vi "SW_Fire_TTL_during_calibration_2.vi"(8 "error in (no error)":errorcluster, 9 "VISA resource in":refnum<visa-resource-name>="Tracker", 10 "Port to fire":u16(ring)=1 items=["Out 1"=1, "Out 2"=2, "Out 3"=4, "Out 4"=8], 11 "TTL pulse length, ms":dbl=250.0 format="%#_13g") -> (0 "error out":errorcluster, 1 "VISA resource out":refnum<visa-resource-name>="Tracker", 3 "Time spent to process command, ms":dbl)   [LabVIEW 2018, in "Tracker.lvlib"]
doc: "Fires TTL High to the TTL2 output for ~250 ms (default)."
uses:
  Tracker.lvlib
  <vilib>/Instr/_visa.llb/VISA Flush IO Buffer Mask.ctl
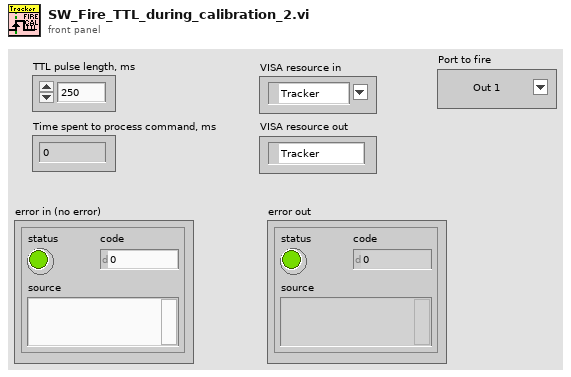
[diagram p1: front panel]
types:
  T1 = typedef "VISA Flush IO Buffer Mask.ctl" = u16
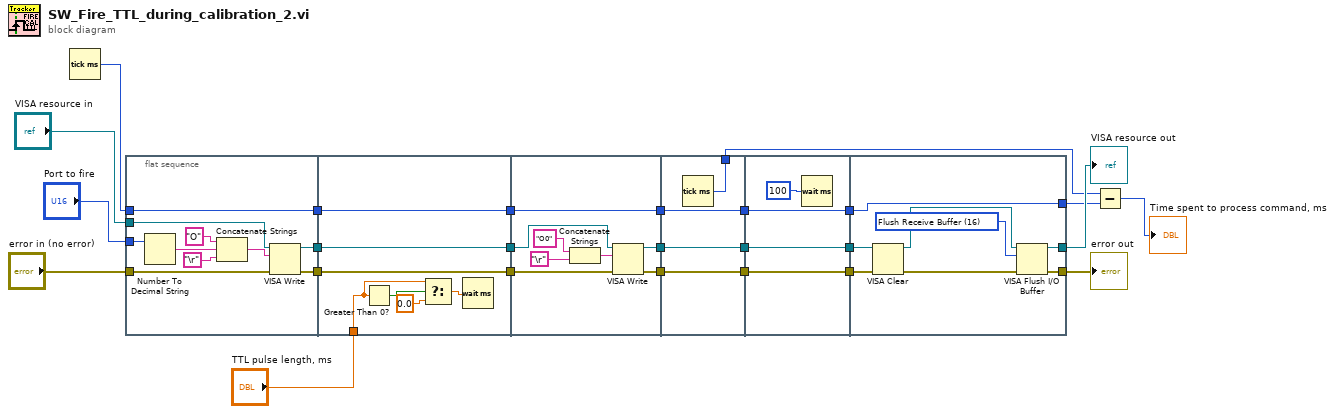
[diagram p0: block diagram]
diagram:
  n1 = Tick Count (ms)() -> (millisecond timer value=w15:u32)
  n2 = flat-sequence {
    tunnel: "VISA resource in" -> [w33]
    tunnel: [w35] -> w21
    tunnel: [w34] -> w20
    tunnel: [w32] -> w19
    tunnel: w15 -> [w32]
    tunnel: "error in (no error)" -> [w31]
    tunnel: "Port to fire" -> [w28]
    tunnel: [w42] -> w16
    tunnel: w21 -> [w42]
    tunnel: [w41] -> w17
    tunnel: w20 -> [w41]
    tunnel: w19 -> [w37]
    tunnel: [w37] -> w18
    tunnel: "TTL pulse length, ms" -> [w36]
    tunnel: w18 -> [w50]
    tunnel: w17 -> [w49]
    tunnel: w16 -> [w48]
    tunnel: [w50] -> w7
    tunnel: [w44] -> w5
    tunnel: [w43] -> w3
    tunnel: w7 -> [w54]
    tunnel: [w54] -> w6
    tunnel: w5 -> [w53]
    tunnel: [w53] -> w4
    tunnel: w3 -> [w52]
    tunnel: [w52] -> w2
    tunnel: [w51] -> w1
    tunnel: w6 -> [w58]
    tunnel: [w58] -> w10
    tunnel: w4 -> [w57]
    tunnel: [w57] -> w9
    tunnel: w2 -> [w56]
    tunnel: [w56] -> w8
    tunnel: [w60] -> w23
    tunnel: [w59] -> w25
    tunnel: [w66] -> w14
    tunnel: w10 -> [w66]
    tunnel: w9 -> [w62]
    tunnel: w8 -> [w61]
    frame #0 {
      n3 = Number To Decimal String(number=w28) -> (decimal integer string=w30:string)  [unwired: 1 in]
      n4 = Concatenate Strings("O" ("string"), w30, "\r") -> (w27:string)
      n5 = VISA Write(VISA resource name=w33, write buffer=w27, error in (no error)=w31) -> (VISA resource name out=w35:refnum<visa-resource-name>, error out=w34:errorcluster)  [unwired: 1 out]
    }
    frame #1 {
      n6 = Greater Than 0?(x=w36) -> (x > 0?=w40:bool)
      n7 = Select(t=w36, s=w40, f=0.0) -> (s? t:f=w39:dbl)
      n8 = Wait (ms)(milliseconds to wait=w39) -> ()  [unwired: 1 out]
    }
    frame #2 {
      n9 = Concatenate Strings("O0" ("write buffer"), "\r") -> (w45:string)
      n10 = VISA Write(VISA resource name=w48, write buffer=w45, error in (no error)=w49) -> (VISA resource name out=w43:refnum<visa-resource-name>, error out=w44:errorcluster)  [unwired: 1 out]
    }
    frame #3 {
      n11 = Tick Count (ms)() -> (millisecond timer value=w51:u32)
    }
    frame #4 {
      n12 = Wait (ms)(milliseconds to wait=u32 100) -> ()  [unwired: 1 out]
    }
    frame #5 {
      w63 = T1 16 items=["Flush Receive Buffer"=16, "Write Transmit Buffer to Device"=32, "Flush Receive Buffer (No I/O)"=64, "Flush Transmit Buffer"=128] ("Mask")
      n13 = VISA Clear(VISA resource name=w61, error in (no error)=w62) -> (VISA resource name out=w65:refnum<visa-resource-name>, error out=w64:errorcluster)
      n14 = VISA Flush I/O Buffer(VISA resource name=w65, mask (16)=w63, error in (no error)=w64) -> (VISA resource name out=w59:refnum<visa-resource-name>, error out=w60:errorcluster)
    }
  }
  n15 = Subtract(x=w1, y=w14) -> (x-y=→"Time spent to process command, ms":u32)
  "VISA resource out" <- w25
  "error out" <- w23
